vi "FactoryMethod.vi"(8 "error in (no error)":errorcluster, 11 "ConcreteCreatorA in":refnum<class "ConcreteCreatorB.lvclass">) -> (0 "error out":errorcluster, 2 "Product.":refnum<class "Product.lvclass">, 3 "ConcreteCreatorA out":refnum<class "ConcreteCreatorB.lvclass">)   [LabVIEW 2020, in "FactoryMethod.lvlib" / "ConcreteCreatorB.lvclass"]
uses:
  ConcreteCreatorB.lvclass
  Product/Product.lvclass
  ConcreteProductB/ConcreteProductB.lvclass
  E:/GitHub/Design-Patterns-GoF_-_NI-LV/Creational/FactoryMethod/Base_Example/ConcreteCreatorB/Product/Product.lvclass
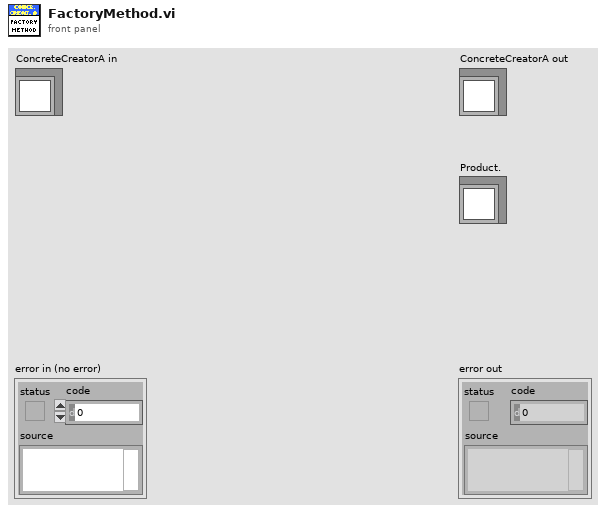
[diagram p1: front panel]
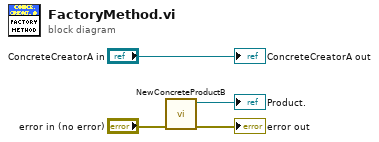
[diagram p0: block diagram]
diagram:
  n1 = call "NewConcreteProductB.vi"("error in (no error)"="error in (no error)") -> ("error out"=→"error out":errorcluster, "ConcreteProductA out"=→"Product.":refnum<class "ConcreteProductB.lvclass">)  [unwired: 9 in]
  "ConcreteCreatorA out" <- "ConcreteCreatorA in"
